vi "destroy.vi"(8 "error in (no error)":errorcluster, 11 "ITaskStopMechanism in":refnum<class "ITaskChannel.lvclass">) -> (0 "error out":errorcluster, 3 "ITaskStopMechanism out":refnum<class "ITaskChannel.lvclass">)   [LabVIEW 2023, in "TLC_Daemon.lvlib" / "ITaskChannel.lvclass"]
doc: "Destroy procedure"
uses:
  ITaskChannel.lvclass
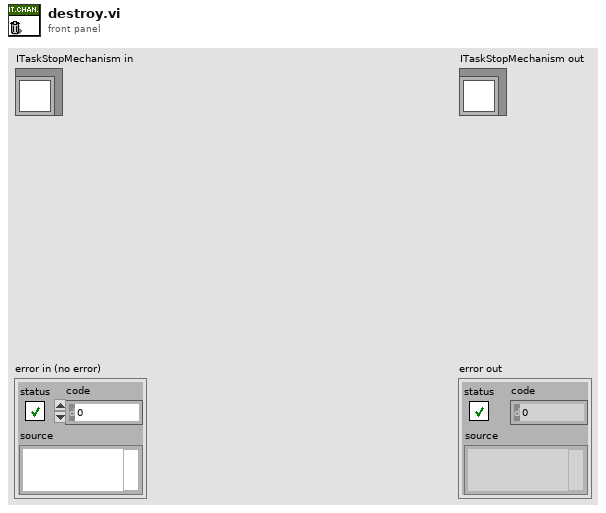
[diagram p1: front panel]
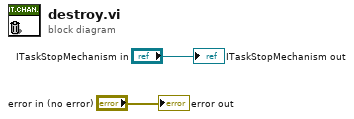
[diagram p0: block diagram]
diagram:
  "error out" <- "error in (no error)"
  "ITaskStopMechanism out" <- "ITaskStopMechanism in"
